vi "LcWebView_AlertDialog_Custom A custom positioned dialog.vi"() -> ()   [LabVIEW 2018, in "LcWebView.lvclass"]
uses:
  LcWebView.lvclass
  webui/ctrls/IconTypeDef.ctl
  webui/ctrls/PositionedDialogType.ctl
  C:/Program Files/National Instruments/LabVIEW 2020/user.lib/_LabVIEWCommon/LcWebView/LcWebView_class/data/Microsoft.Web.WebView2.WinForms.dll
panel:
  out "BrowserProcessId":u32
  in  "stop":bool
  out "Result":string
  out "Status Message":string
  in  "Web":refnum<k24>(container)
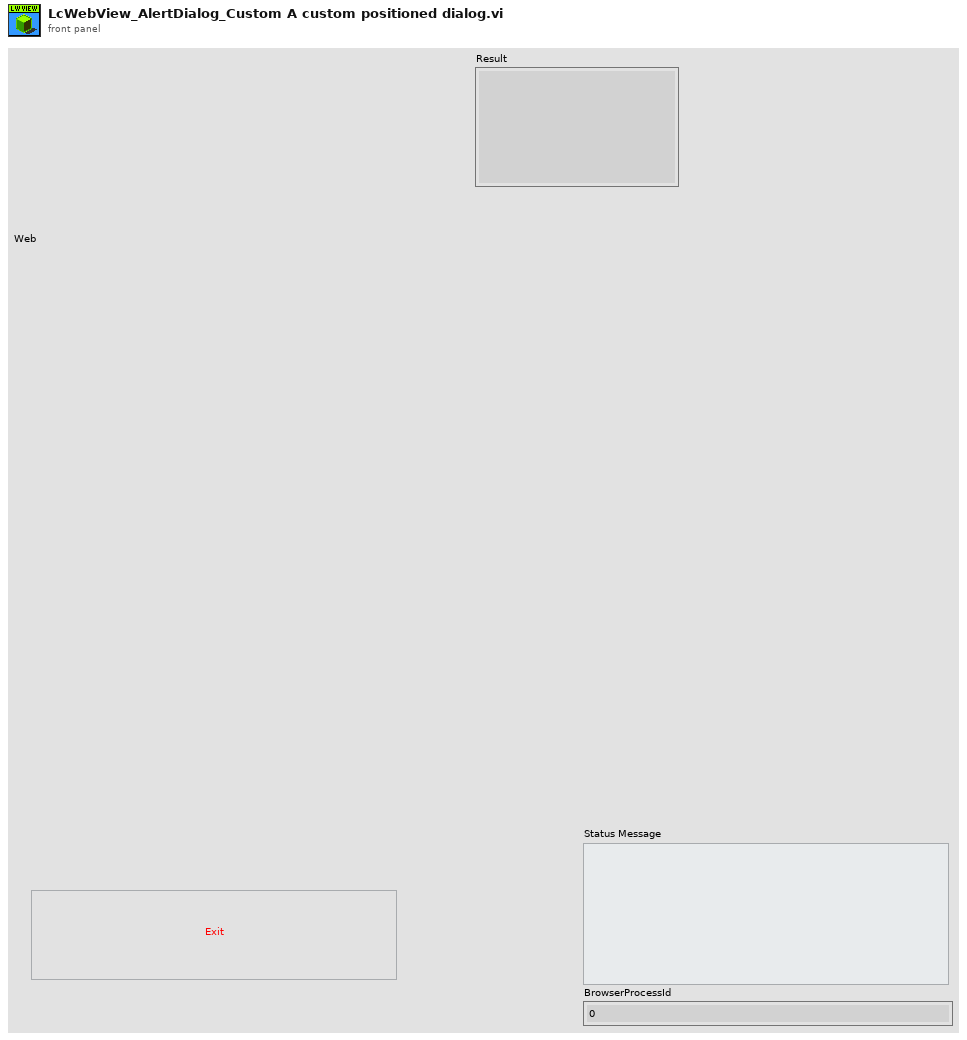
[diagram p1: front panel]
types:
  T1 = typedef "LcWebView.lvclass/IconTypeDef.ctl" = enum16{"success", "error", "warning", "info", "question"}
  T2 = typedef "LcWebView.lvclass/PositionedDialogType.ctl" = cluster{"title":string, "showConfirmButton":bool, "position":string, "timer":dbl, "icon":T1}
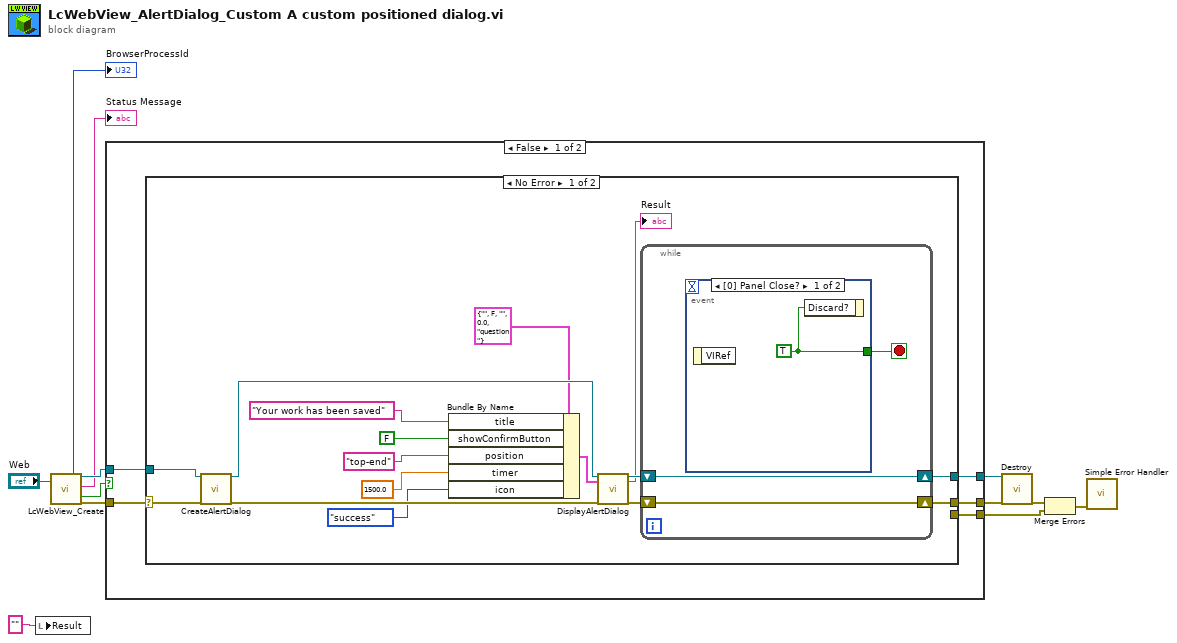
[diagram p0: block diagram]
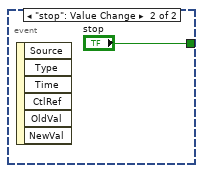
[diagram p2: hidden frame]
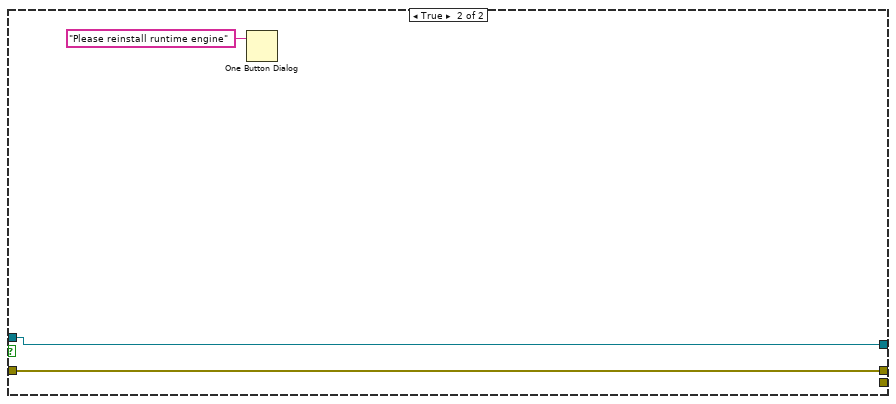
[diagram p4: hidden frame]
diagram:
  n1 = local write "Result"("" ("Result")) -> ()
  n2 = call "LcWebView_Create.vi"("Webview container"="Web") -> ("BrowserProcessId"=→"BrowserProcessId":u32, "reference out"=w11:refnum<class "LcWebView.lvclass">, "Status Message"=→"Status Message":string, "Reinstall Runtime"=w4:bool, "Error Out"=w10:errorcluster)  [unwired: 11 in, 3 out]
  n3 = case shown="False" w4 {
    tunnel: w11 -> [w17 w43]
    tunnel: w10 -> [w16 w42]
    tunnel: [w15 w43] -> w9
    tunnel: [w13 w42] -> w8
    tunnel: [w14 _] -> w5
    frame False {
      n4 = case shown="No Error" w16 {
        selector: w16 -> [w30 w39]
        tunnel: w17 -> [w31 w40]
        tunnel: [w32 w40] -> w15
        tunnel: [w33 _] -> w13
        tunnel: [_ w39] -> w14
        frame No Error {
          n5 = call-dynamic "CreateAlertDialog.vi"("reference in"=w31, "Error In"=w30) -> ("reference out"=w29:refnum<class "LcWebView.lvclass">, "Error Out"=w28:errorcluster)  [unwired: 16 in]
          n6 = Bundle By Name(cluster=T2 {"title"="", "showConfirmButton"=FALSE, "position"="", "timer"=0.0, "icon"=enum."question"}, "title"="Your work has been saved", "showConfirmButton"=FALSE ("showDenyButton"), "position"="top-end" ("confirmButtonText"), "timer"=1500.0, "icon"=IconTypeDef."success" ("Icon")) -> (w25:T2)
          n7 = call-dynamic "DisplayAlertDialog.vi"("reference in"=w29, "Message"=w25, "Error In"=w28) -> ("reference out"=w27:refnum<class "LcWebView.lvclass">, "Result"=→"Result":string, "Error Out"=w26:errorcluster)  [unwired: 14 in]
          n8 = while {
            shift-right: [w36] -> w32
            shift-left: w27 -> [w36]
            shift-right: [w35] -> w33
            shift-left: w26 -> [w35]
            stop <- w34 stop-if-true
            n9 = event shown="[0] Panel Close?" {
              selector: _ -> [_ _]
              dyn-events: _ -> [_ _]
              timeout: _ -> [_ _]
              tunnel: [w37 "stop"] -> w34
              event Panel Close? {
                w37 = TRUE ("Discard?")
                n10 = event-data() -> ()  [unwired: 1 in, 1 out]
                n11 = event-data("Discard?"=w37) -> ()  [unwired: 1 in, 1 out]
              }
              event "stop": Value Change {
                n12 = event-data() -> ()  [unwired: 1 in, 6 out]
              }
            }
          }
        }
        frame Error {
        }
      }
    }
    frame True {
      n13 = One Button Dialog(message="Please reinstall runtime engine") -> ()  [unwired: 1 in, 1 out]
    }
  }
  n14 = call-dynamic "Destroy.vi"("reference in"=w9, "Error In"=w8) -> ("Error Out"=w7:errorcluster)  [unwired: 16 in, 1 out]
  n15 = Merge Errors(w7, w5) -> (w2:errorcluster)
  n16 = call <vilib>:"Simple Error Handler.vi"("error in (no error)"=w2) -> ()  [unwired: 4 in, 5 out]
